vi "Respond.vi"(7 "Sender is Waiting?(F)":bool, 8 "error in (no error)":errorcluster, 9 "Data":refnum<class "Data.lvclass">, 10 "Actor in":refnum<class "Actor.lvclass">, 11 "Response Core in":refnum<class "Response Core.lvclass">) -> (0 "error out":errorcluster, 2 "Actor out":refnum<class "Actor.lvclass">)   [LabVIEW 2020, in "Publisher.lvlib" / "Response Core.lvclass"]
doc: "Handle the Data Action response.\n\nThe default drops the response core and does nothing else."
uses:
  Response Core.lvclass
  PPL/HDH.Data.Generic.lvlibp/Data.lvclass
  PPL/HDH.Actor Framework.Core.Actor.lvlibp/1abvi3w/vi.lib/ActorFramework/Actor/Actor.lvclass
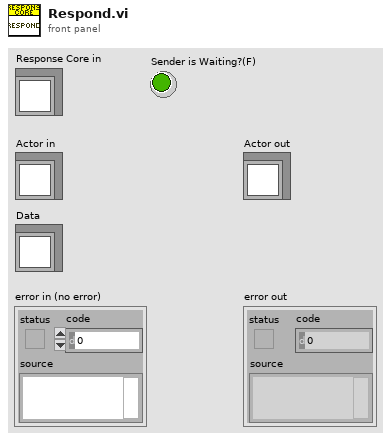
[diagram p1: front panel]
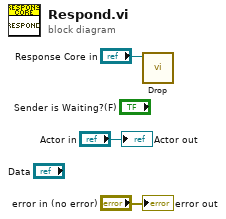
[diagram p0: block diagram]
diagram:
  n1 = call-dynamic "Drop.vi"("Response Core in"="Response Core in") -> ()  [unwired: 11 in]
  "error out" <- "error in (no error)"
  "Actor out" <- "Actor in"
